vi "XML_Save_File.vi"(8 "error in (no error)":errorcluster caption="错误输入（无错误）", 10 "UUT OUT Data":string[][](array[string]), 11 "XML File Path":path caption="XML文件路径") -> (0 "error out":errorcluster caption="错误输出", 2 "XML String":string caption="XML字符串", 3 "XML File Path(duplicate)":path caption="XML文件路径（副本）")   [LabVIEW 2018]
uses:
  Global.vi
panel:
  out "字符串":string
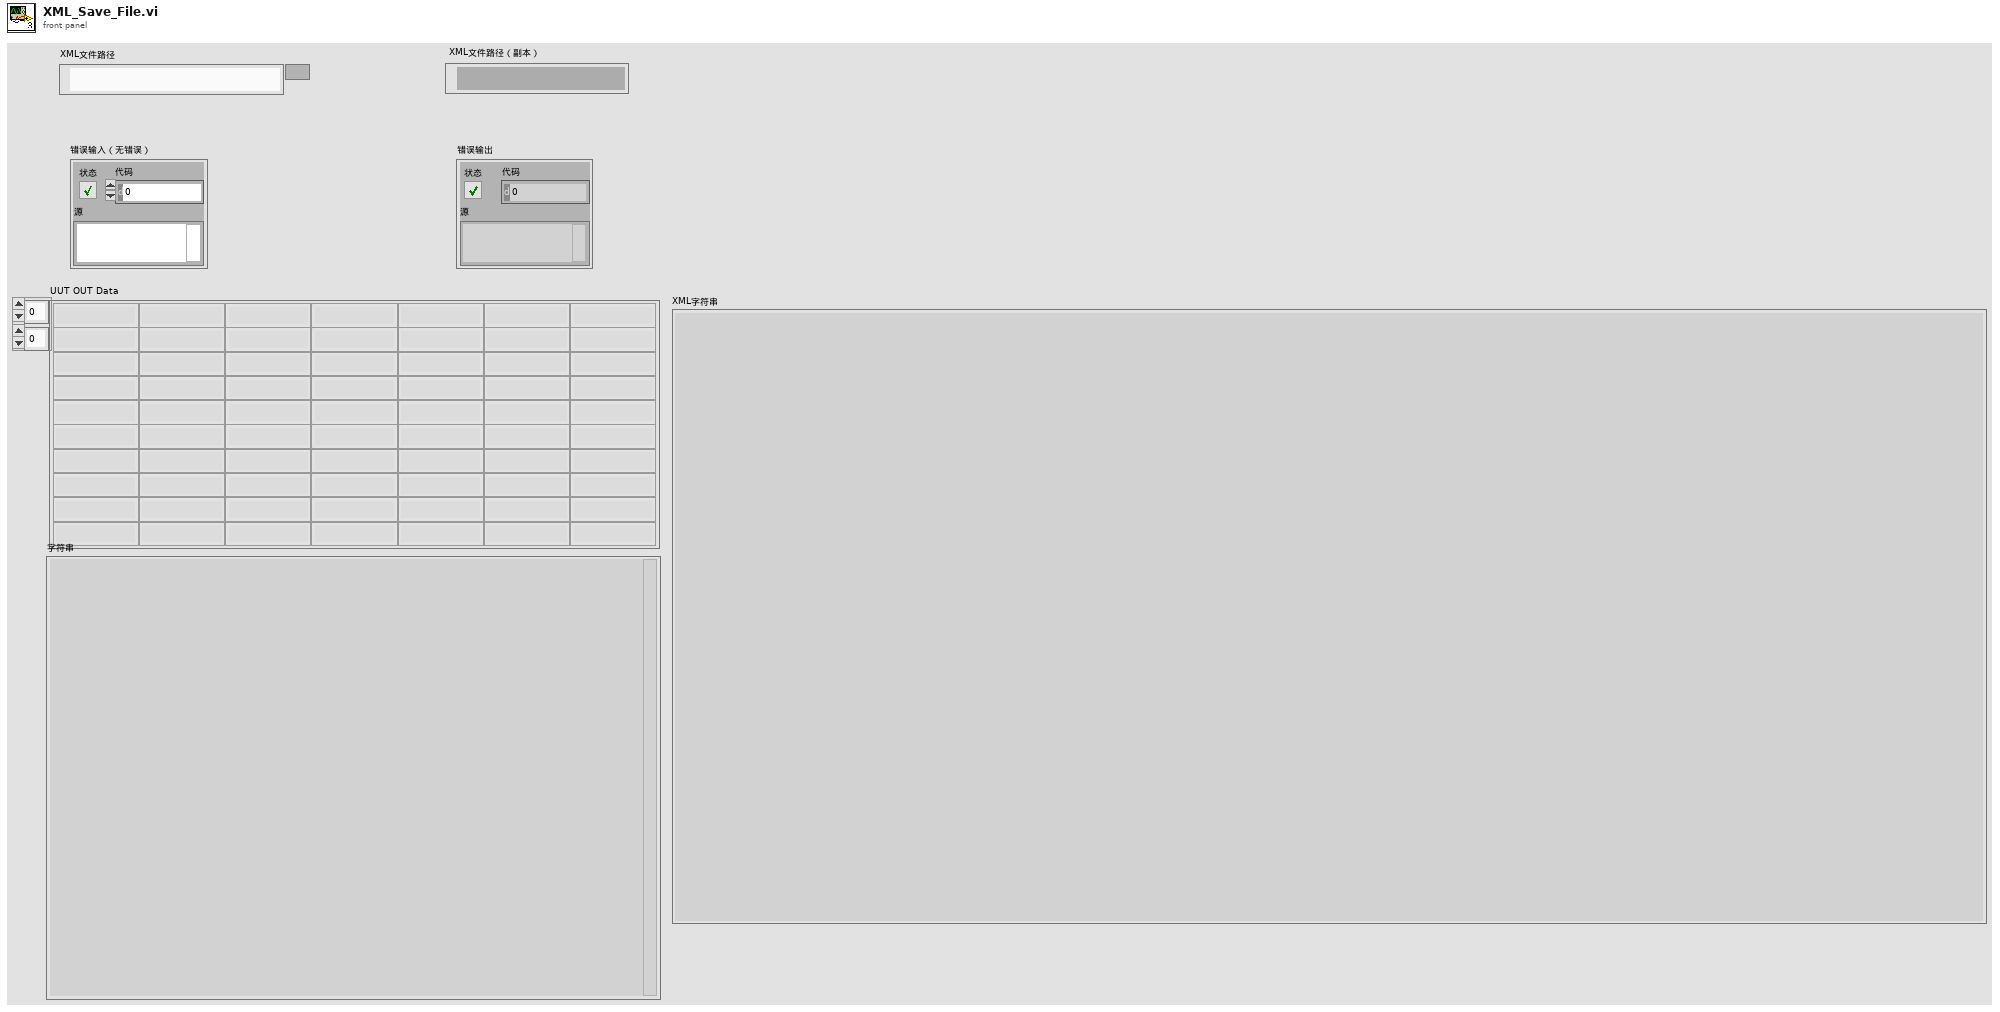
[diagram p1: front panel]
types:
  T1 = cluster{"Unit Timestamp":string, "SerialNumber":string, "StatusCode":string, "DateTimeStart":string, "DateTimeEnd":string, "TestProgramVersion":string, "TestFixtureNumber":string}
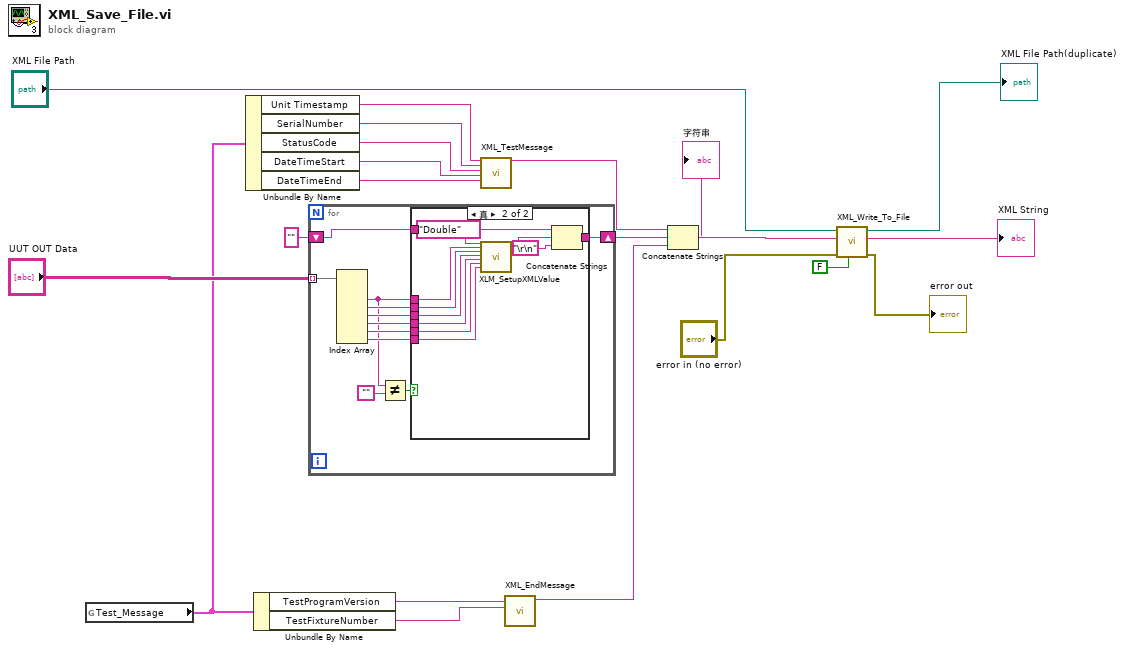
[diagram p0: block diagram]
diagram:
  n1 = global read "Global.vi" "Test_Message"() -> (w10:T1)
  n2 = Unbundle By Name(w10) -> ("Unit Timestamp"=w9:string, "SerialNumber"=w8:string, "StatusCode"=w7:string, "DateTimeStart"=w6:string, "DateTimeEnd"=w5:string)
  n3 = Unbundle By Name(w10) -> ("TestProgramVersion"=w12:string, "TestFixtureNumber"=w11:string)
  n4 = for {
    tunnel: "UUT OUT Data" -> [w31] mode=indexing
    shift-right: [w30] -> w17
    shift-left: "" -> [w29]
    n5 = Index Array(array=w31) -> (element #2=w22:string, element #3=w28:string, element #4=w27:string, element #5=w26:string, element #6=w25:string, element #7=w24:string)  [unwired: 7 in, 1 out]
    n6 = Not Equal?(x=w22, y="") -> (x != y?=w21:bool)
    n7 = case shown="真" w21 {
      tunnel: [w32 w43] -> w30
      tunnel: w29 -> [w32 w42]
      tunnel: w22 -> [_ w39]
      tunnel: w28 -> [_ w38]
      tunnel: w27 -> [_ w37]
      tunnel: w26 -> [_ w36]
      tunnel: w25 -> [_ w35]
      tunnel: w24 -> [_ w34]
      frame False {
      }
      frame True {
        n8 = call "XLM_SetupXMLValue.vi"("ValueUnit"="Double", "Name"=w39, "Max"=w38, "Value"=w37, "Min"=w36, "Uint"=w35, "Status"=w34) -> ("生成的XML 2"=w40:string)  [unwired: 20 in]
        n9 = Concatenate Strings(w42, w40, "\r\n") -> (w43:string)
      }
    }
  }
  "字符串" <- w17
  n10 = call "XML_TestMessage.vi"("Unit Timestamp"=w9, "SerialNumber"=w8, "StatusCode"=w7, "DateTimeStart"=w6, "DateTimeEnd"=w5) -> ("连接的字符串"=w16:string)  [unwired: 13 in, 1 out]
  n11 = call "XML_EndMessage.vi"("TestFixtureNumber"=w11, "TestProgramVersion"=w12) -> ("连接的字符串"=w15:string)  [unwired: 9 in]
  n12 = Concatenate Strings(w16, w17, w15) -> (w18:string)
  n13 = call "XML_Write_To_File.vi"("Standalone? (T)"=FALSE, "error in (no error)"="error in (no error)", "XML Input"=w18, "XML File Path"="XML File Path") -> ("error out"=→"error out":errorcluster, "XML String"=→"XML String":string, "XML File Path(duplicate)"=→"XML File Path(duplicate)":path)  [unwired: 5 in]
